vi "DuplicateNode.vi"(7 "same parent?":bool, 8 "error in":errorcluster, 10 "new parent":T1, 11 "node ref in":T1) -> (0 "error out":errorcluster, 3 "new node ref":T1)   [LabVIEW 2013, in "NISE_CEF_TreeControl.lvlib"]
doc: "This VI duplicates a creates duplicate of a node.\nIf same parent is set to true the new node will use current parent, if set to false it will be added to the parent specified in the new parent terminal"
uses:
  NISE_CEF_TreeControl.lvlib
  Node/NodeRef.ctl
  Node/NISE_CEF_Node.lvclass
  Node/NISE_CEF_Node.lvclass/NISE_CEF_Node.ctl
  Node/ReadParent.vi
  Node/ReadChildren.vi
  Node/WriteChildren.vi
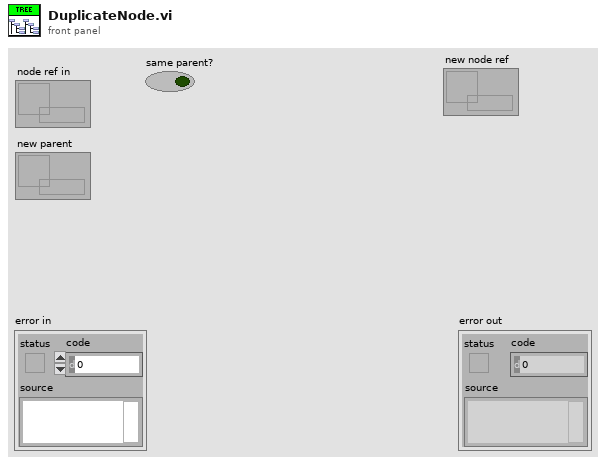
[diagram p1: front panel]
types:
  T1 = typedef "NISE_CEF_Node.lvclass/NodeRef.ctl" = refnum<data-value>
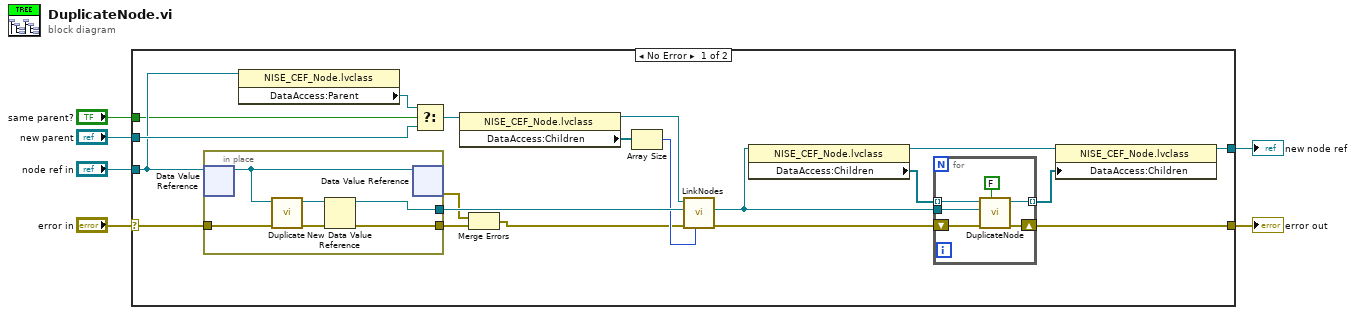
[diagram p0: block diagram]
diagram:
  n1 = case shown="No Error" "error in" {
    selector: "error in" -> [w15 w39]
    tunnel: [w24 w39] -> w5
    tunnel: "node ref in" -> [w22 _]
    tunnel: [w16 _] -> w3
    tunnel: "new parent" -> [w26 _]
    tunnel: "same parent?" -> [w10 _]
    frame No Error {
      n2 = in-place {
        in-place-border: [w38] -> w21
        in-place-border: w15 -> [w35]
        in-place-border: [w33] -> w8
        n3 = in-place-dvr #1(w22) -> (w37:refnum<class "NISE_CEF_Node.lvclass">)  [unwired: 1 out]
        n4 = call-dynamic "Duplicate.vi"("error in"=w35, "node in"=w37) -> ("error out"=w34:errorcluster, "node copy out"=w36:refnum<class "NISE_CEF_Node.lvclass">)  [unwired: 8 in]
        n5 = New Data Value Reference(data value=w36, error in=w34) -> (data value reference=w38:refnum<data-value>, error out=w33:errorcluster)
        n6 = in-place-dvr #1(w37) -> (w9:errorcluster)  [unwired: 1 out]
      }
      n7 = property class="NISE_CEF_Node.lvclass"(reference=w22) -> ("DataAccess:Parent"=w23:T1)  [unwired: 1 in, 2 out]
      n8 = Select(t=w23, s=w10, f=w26) -> (s? t:f=w14:T1)
      n9 = property class="NISE_CEF_Node.lvclass"(reference=w14) -> (reference out=w13:T1, "DataAccess:Children"=w12:T1[])  [unwired: 1 in, 1 out]
      n10 = Merge Errors(w9, w8) -> (w7:errorcluster)
      n11 = Array Size(array=w12) -> (size(s)=w11:i32)
      n12 = call "LinkNodes.vi"("index"=w11, "error in"=w7, "child in"=w21, "parent in"=w13) -> ("error out"=w25:errorcluster, "child out"=w17:T1)  [unwired: 5 in, 1 out]
      n13 = property class="NISE_CEF_Node.lvclass"(reference=w17) -> (reference out=w20:T1, "DataAccess:Children"=w19:T1[])  [unwired: 1 in, 1 out]
      n14 = for {
        tunnel: w19 -> [w32] mode=indexing
        tunnel: [w31] -> w18 mode=indexing
        tunnel: w17 -> [w30]
        shift-right: [w28] -> w24
        shift-left: w25 -> [w29]
        n15 = call "DuplicateNode.vi"("same parent?"=FALSE ("s"), "error in"=w29, "new parent"=w30, "node ref in"=w32) -> ("error out"=w28:errorcluster, "new node ref"=w31:T1)  [unwired: 6 in]
      }
      n16 = property class="NISE_CEF_Node.lvclass"(reference=w20, "DataAccess:Children"=w18) -> (reference out=w16:T1)  [unwired: 1 in, 1 out]
    }
    frame Error {
    }
  }
  "error out" <- w5
  "new node ref" <- w3
